vi "generate-analog-out-multiple-channels-save.vi"(11 "error in":errorcluster) -> (15 "error out":errorcluster)   [LabVIEW 2020]
uses:
  <vilib>/Utility/error.llb/DialogType.ctl
  <vilib>/DAQmx/write.llb/DAQmx Write (Analog 1D Wfm NChan NSamp).vi
  <vilib>/DAQmx/create/channels.llb/DAQmx Create Channel (AO-Voltage-Basic).vi
  <vilib>/DAQmx/configure/timing.llb/DAQmx Timing (Use Waveform).vi
  <vilib>/DAQmx/miscellaneous.llb/DAQmx Fill In Error Info.vi
  <vilib>/Utility/file.llb/Read Delimited Spreadsheet (string).vi
panel:
  out "Waveform Array Out":waveform(dbl)[](array[waveform])
  in  "t0":timestamp
  in  "dt":dbl
  out "New t0":timestamp
  out "Array 4":dbl[][](array[numeric])
  out "Array 3":dbl[][](array[numeric])
  out "Y":dbl[][](array[numeric])
  out "all rows of data":string[][](array[string])
  out "subarray":dbl[](array[numeric])
  in  "Array":dbl[][](array[numeric])
  out "Waveform Chart 2":waveform(dbl)(graph)
  out "Waveform Chart 1":waveform(dbl)(graph)
  out "Waveform Chart All":waveform(dbl)[](graph)
  in  "Delta T":dbl=0.0005
  in  "stop":bool
  in  "Physical Channel CH0 (Virtual)":tag="DAQ1/ao0"
  in  "physical Output CH1 (Virtual)":tag="DAQ1/ao0"
  in  "EMG Data File":path=path "C:/data/new-4rows-4columns.csv"
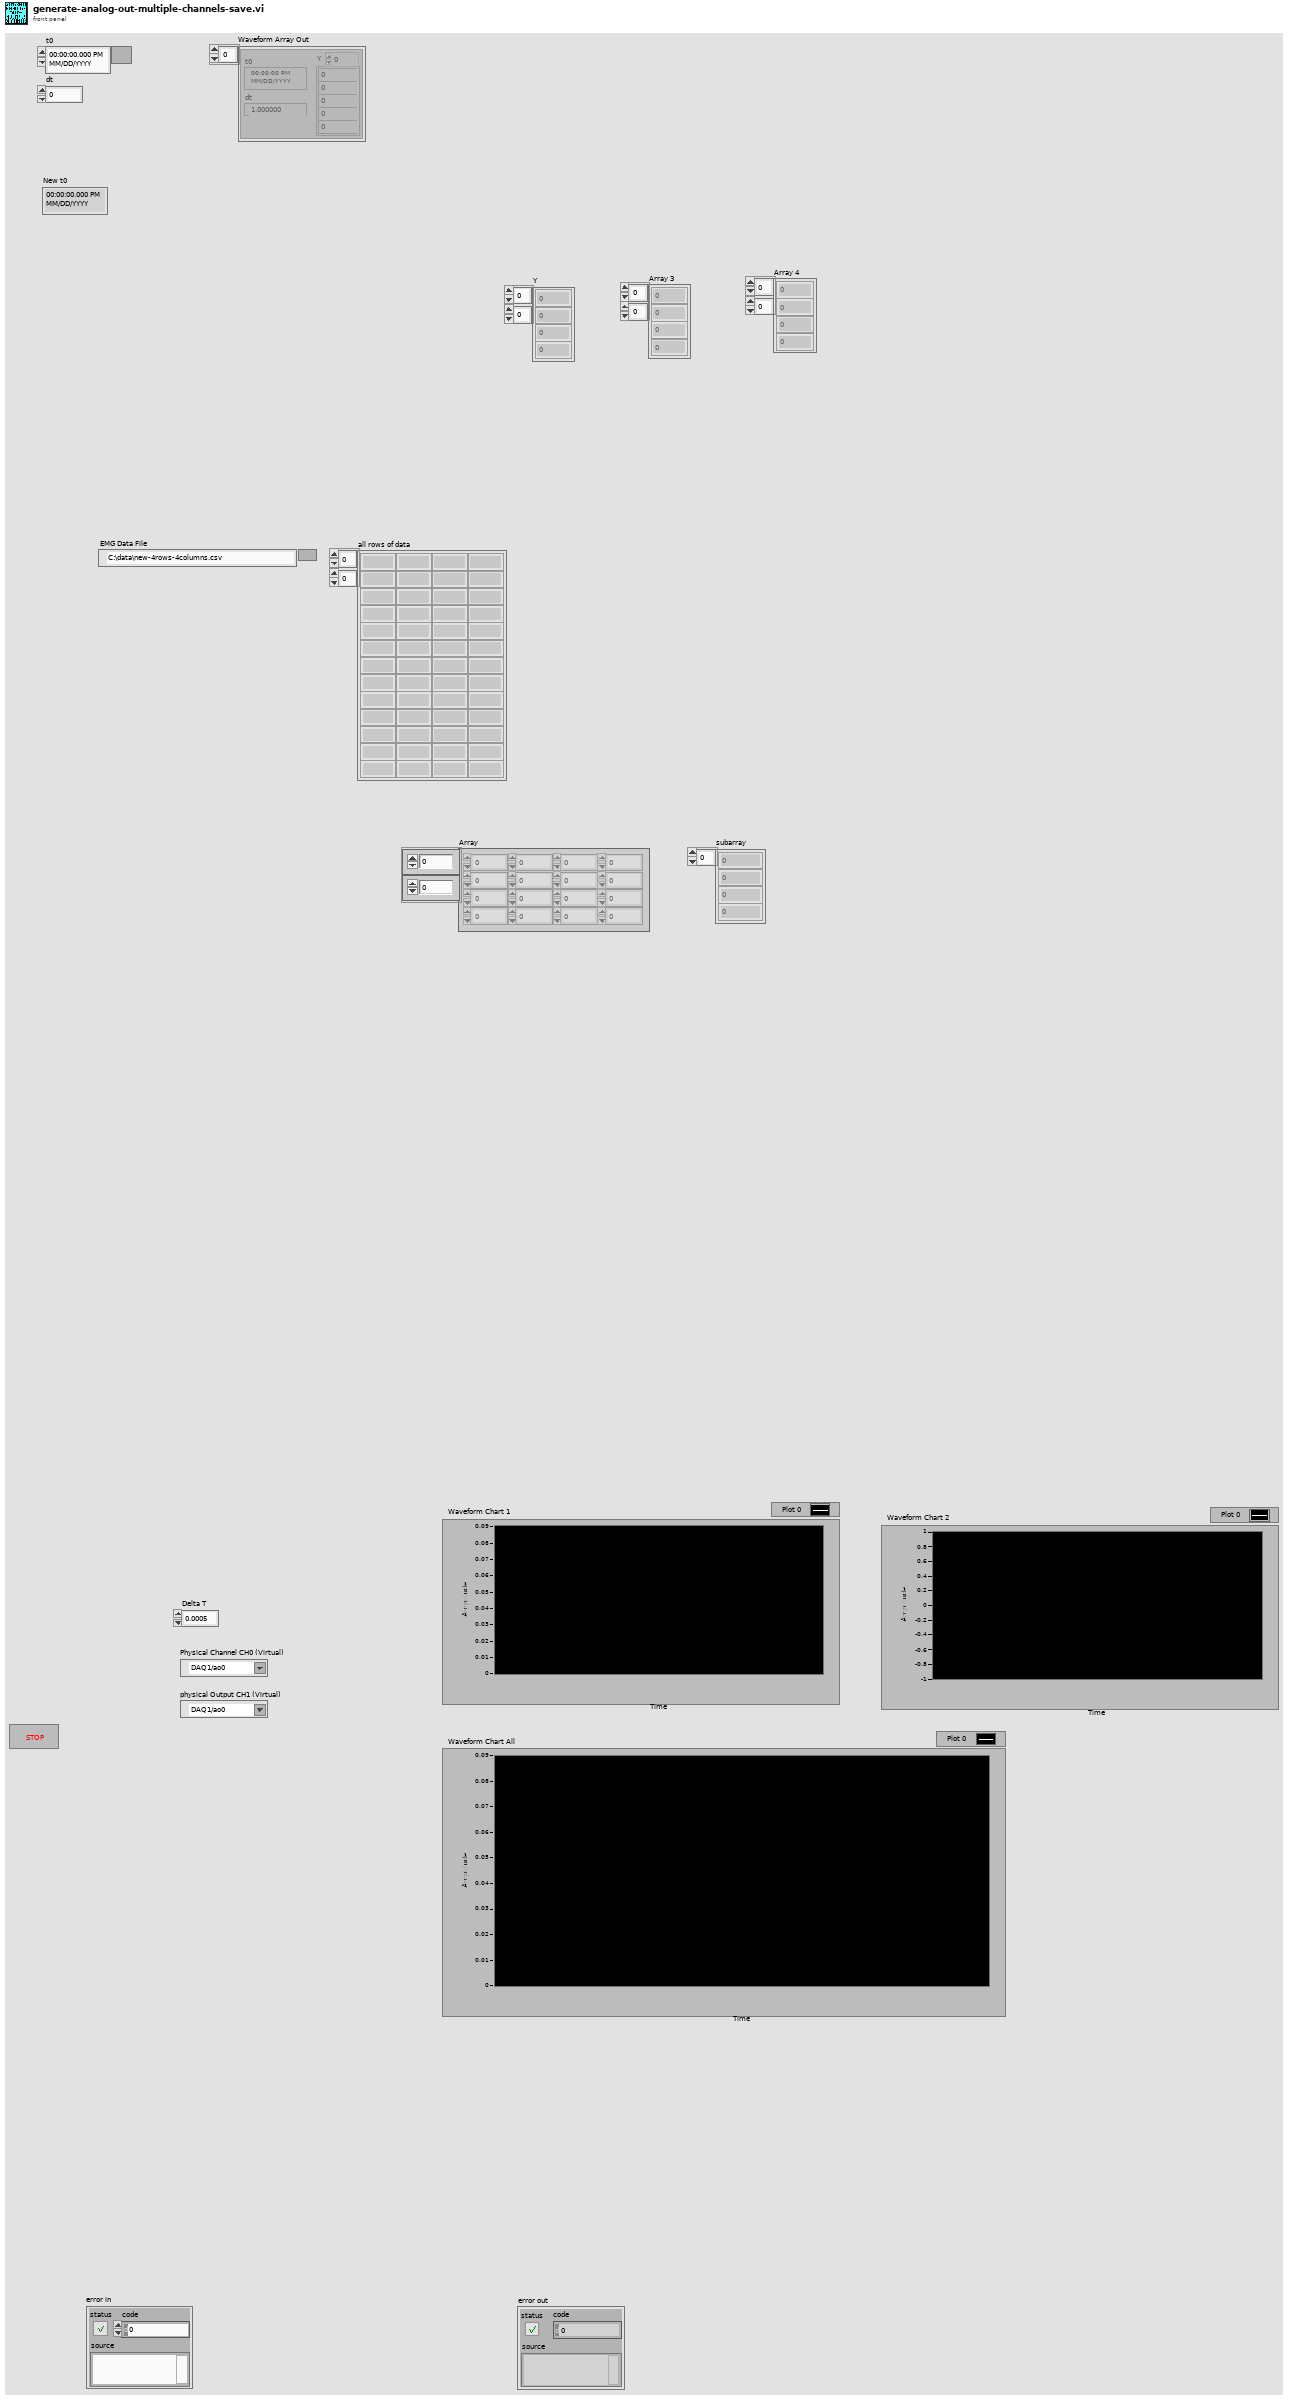
[diagram p1: front panel]
types:
  T1 = typedef "DialogType.ctl" = u16
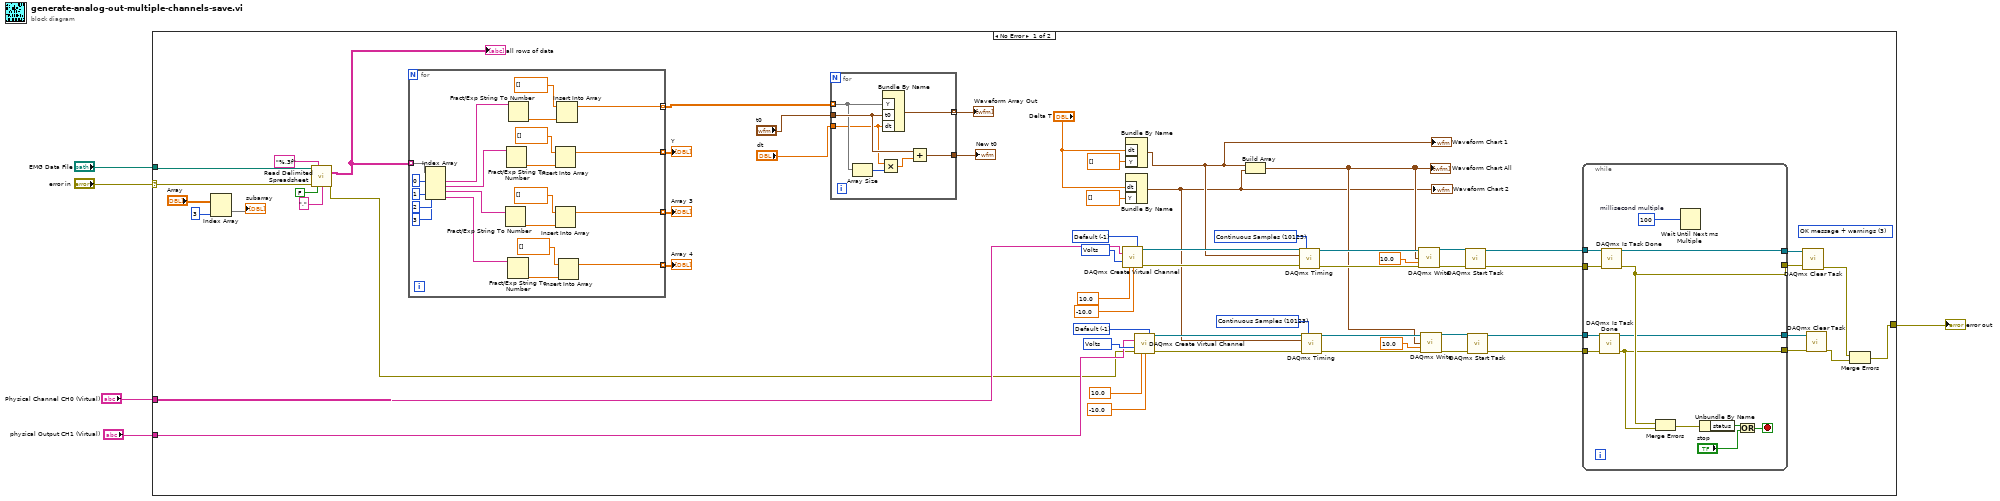
[diagram p0: block diagram]
diagram:
  n1 = case shown="No Error" "error in" {
    selector: "error in" -> [w17 w108]
    tunnel: [w44 w108] -> w4
    tunnel: "EMG Data File" -> [w22 _]
    tunnel: "Physical Channel CH0 (Virtual)" -> [w39 _]
    tunnel: "physical Output CH1 (Virtual)" -> [w32 _]
    frame No Error {
      w33 = 10348 items=["Volts"=10348, "From Custom Scale"=10065] ("units")
      w34 = -1 items=["Default"=-1, "RSE"=10083, "Differential"=10106, "Pseudodifferential"=12529] ("output terminal configuration")
      w40 = 10348 items=["Volts"=10348, "From Custom Scale"=10065] ("units")
      w41 = -1 items=["Default"=-1, "RSE"=10083, "Differential"=10106, "Pseudodifferential"=12529] ("output terminal configuration")
      w57 = 10123 items=["Finite Samples"=10178, "Continuous Samples"=10123] ("sample mode")
      (unwired) T1 3 items=["no dialog", "OK message", "continue or stop message", "OK message + warnings", "continue/stop + warnings"] ("type of dialog (OK msg:1)")
      w66 = 10123 items=["Finite Samples"=10178, "Continuous Samples"=10123] ("sample mode")
      n2 = Index Array(array="Array", index (col)=3 ("disabled index (col)")) -> (element=→"subarray":dbl[])  [unwired: 1 in]
      n3 = call-poly <vilib>:"Read Delimited Spreadsheet.vi"("file path (dialog if empty)"=w22, "format (%s)"="%.3f" ("format (%.3f)"), "error in (no error)"=w17, "transpose? (F)"=FALSE, "delimiter (\\t)"="," ("delimiter (\\t)")) -> ("all rows"=w16:string[][], "error out"=w18:errorcluster)  [unwired: 5 in, 4 out]
      "all rows of data" <- w16
      n4 = for {
        tunnel: w16 -> [w94] mode=indexing
        tunnel: [w88] -> w6 mode=indexing
        tunnel: [w79] -> w14 mode=indexing
        tunnel: [w78] -> w13 mode=indexing
        tunnel: [w75] -> w12 mode=indexing
        n5 = Index Array(array=w94, index #1=0 ("index"), index #2=1 ("index"), index #3=2 ("index"), index #4=3 ("index")) -> (element #1=w86:string, element #2=w81:string, element #3=w80:string, element #4=w74:string)
        n6 = Fract/Exp String To Number(string=w80) -> (number=w83:dbl)  [unwired: 3 in, 1 out]
        n7 = Fract/Exp String To Number(string=w81) -> (number=w85:dbl)  [unwired: 3 in, 1 out]
        n8 = Fract/Exp String To Number(string=w74) -> (number=w77:dbl)  [unwired: 3 in, 1 out]
        n9 = Fract/Exp String To Number(string=w86) -> (number=w89:dbl)  [unwired: 3 in, 1 out]
        n10 = Insert Into Array(array=dbl[] [] ("Y"), new element=w85) -> (w79:dbl[])  [unwired: 1 in]
        n11 = Insert Into Array(array=dbl[] [], new element=w83) -> (w78:dbl[])  [unwired: 1 in]
        n12 = Insert Into Array(array=dbl[] [] ("Y"), new element=w89) -> (w88:dbl[])  [unwired: 1 in]
        n13 = Insert Into Array(array=dbl[] [], new element=w77) -> (w75:dbl[])  [unwired: 1 in]
      }
      "Y" <- w14
      "Array 3" <- w13
      "Array 4" <- w12
      n14 = for {
        tunnel: w6 -> [w71] mode=indexing
        tunnel: [w73] -> w7 mode=indexing
        tunnel: "t0" -> [w72]
        tunnel: "dt" -> [w69]
        tunnel: [w67] -> w10
        n15 = Array Size(array=w71) -> (size(s)=w70:i32)
        n16 = Multiply(x=w69, y=w70) -> (x*y=w68:dbl)
        n17 = Bundle By Name("Y"=w71, "t0"=w72, "dt"=w69) -> (w73:waveform(dbl))  [unwired: 1 in]
        n18 = Add(x=w72, y=w68) -> (x+y=w67:timestamp)
      }
      "Waveform Array Out" <- w7
      "New t0" <- w10
      n19 = call-poly <vilib>:"DAQmx Create Virtual Channel.vi"("maximum value"=10.0 ("Maximum Value"), "minimum value"=-10.0 ("Minimum Value"), "output terminal configuration"=w41, "physical channels"=w39, "units"=w40) -> ("task out"=w38:refnum<k21>, "error out"=w37:errorcluster)  [unwired: 9 in]
      n20 = Bundle By Name("dt"="Delta T", "Y"=dbl[] []) -> (w26:waveform(dbl))  [unwired: 1 in]
      "Waveform Chart 2" <- w26
      n21 = Bundle By Name("dt"="Delta T", "Y"=dbl[] []) -> (w27:waveform(dbl))  [unwired: 1 in]
      "Waveform Chart 1" <- w27
      n22 = call-poly <vilib>:"DAQmx Create Virtual Channel.vi"("maximum value"=10.0 ("Maximum Value"), "minimum value"=-10.0 ("Minimum Value"), "output terminal configuration"=w34, "physical channels"=w32, "units"=w33, "error in"=w18) -> ("task out"=w31:refnum<k21>, "error out"=w30:errorcluster)  [unwired: 8 in]
      n23 = Build Array(w27, w26) -> (w28:waveform(dbl)[])
      "Waveform Chart All" <- w28
      n24 = call-poly <vilib>:"DAQmx Timing.vi"("task/channels in"=w38, "sample mode"=w66, "waveform"=w27, "error in"=w37) -> ("task out"=w61:refnum<k21>, "error out"=w51:errorcluster)  [unwired: 10 in]
      n25 = call-poly <vilib>:"DAQmx Timing.vi"("task/channels in"=w31, "sample mode"=w57, "waveform"=w26, "error in"=w30) -> ("task out"=w53:refnum<k21>, "error out"=w52:errorcluster)  [unwired: 10 in]
      n26 = call-poly <vilib>:"DAQmx Write.vi"("task/channels in"=w61, "data"=w28, "timeout"=10.0 ("Wirite Timeout"), "error in"=w51) -> ("task out"=w65:refnum<k21>, "error out"=w64:errorcluster)  [unwired: 9 in, 1 out]
      n27 = call-poly <vilib>:"DAQmx Write.vi"("task/channels in"=w53, "data"=w28, "timeout"=10.0 ("Wirite Timeout"), "error in"=w52) -> ("task out"=w56:refnum<k21>, "error out"=w55:errorcluster)  [unwired: 9 in, 1 out]
      n28 = call <vilib>:"DAQmx Start Task.vi"("task/channels in"=w65, "error in"=w64) -> ("task out"=w60:refnum<k21>, "error out"=w62:errorcluster)  [unwired: 12 in]
      n29 = call <vilib>:"DAQmx Start Task.vi"("task/channels in"=w56, "error in"=w55) -> ("task out"=w50:refnum<k21>, "error out"=w49:errorcluster)  [unwired: 12 in]
      n30 = while {
        tunnel: w60 -> [w107]
        tunnel: [w106] -> w59
        tunnel: w62 -> [w105]
        tunnel: [w97] -> w58
        tunnel: w50 -> [w100]
        tunnel: w49 -> [w99]
        tunnel: [w96] -> w48
        tunnel: [w95] -> w47
        stop <- w103 stop-if-true
        w104 = u32 100  # millisecond multiple
        n31 = call <vilib>:"DAQmx Is Task Done.vi"("task/channels in"=w100, "error in"=w99) -> ("task out"=w96:refnum<k21>, "error out"=w95:errorcluster)  [unwired: 11 in, 1 out]
        n32 = call <vilib>:"DAQmx Is Task Done.vi"("task/channels in"=w107, "error in"=w105) -> ("task out"=w106:refnum<k21>, "error out"=w97:errorcluster)  [unwired: 11 in, 1 out]
        n33 = Merge Errors(w97, w95) -> (w98:errorcluster)
        n34 = Wait Until Next ms Multiple(millisecond multiple=w104) -> ()  [unwired: 1 out]
        n35 = Unbundle By Name(w98) -> ("status"=w102:bool)
        n36 = Or(x=w102, y="stop") -> (x .or. y?=w103:bool)
      }
      n37 = call <vilib>:"DAQmx Clear Task.vi"("task in"=w59, "error in"=w58) -> ("error out"=w46:errorcluster)  [unwired: 13 in]
      n38 = call <vilib>:"DAQmx Clear Task.vi"("task in"=w48, "error in"=w47) -> ("error out"=w45:errorcluster)  [unwired: 13 in]
      n39 = Merge Errors(w46, w45) -> (w44:errorcluster)
    }
    frame Error {
    }
  }
  "error out" <- w4
